vi "Write.vi"(8 "error in":errorcluster, 10 "ConfigData":T1 {"Inactivity Time" format="%#_g Sec"; "Travel Time" format="%#_g Sec"; "Door Close" format="%#_g Sec"; "Door Open" format="%#_g Sec"}, 11 "Config File In":path) -> (0 "error out":errorcluster, 3 "Config File Out":path)   [LabVIEW 2020, in "ConfigurationDatabase.lvlib"]
doc: "Writes and Save configuration data for the simulated configuration database\n[Covers: CD4]"
uses:
  ConfigurationDatabase.lvlib
  Controls/Configuration Data.ctl
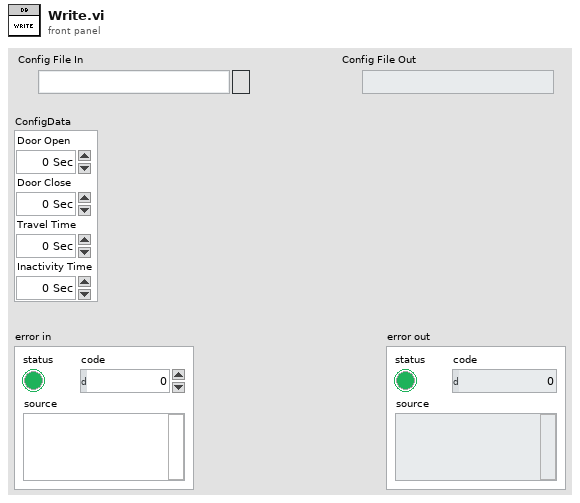
[diagram p1: front panel]
types:
  T1 = typedef "ConfigurationDatabase.lvlib/Configuration Data.ctl" = cluster{"Door Open":dbl, "Door Close":dbl, "Travel Time":dbl, "Inactivity Time":dbl}
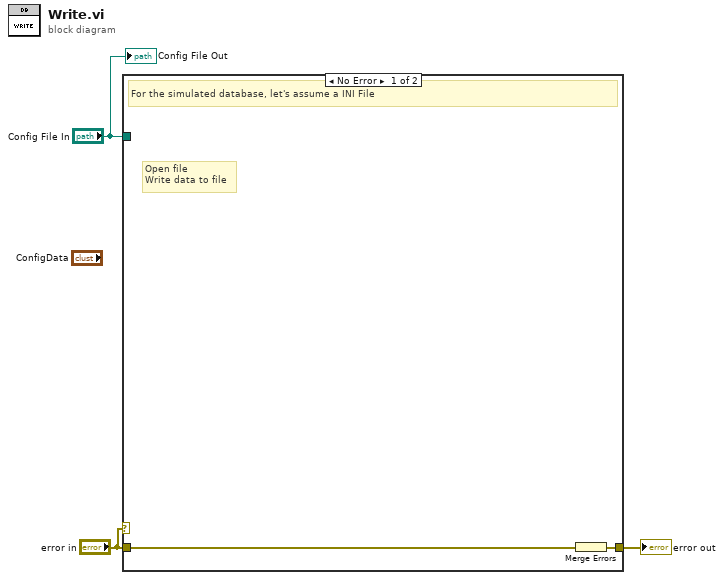
[diagram p0: block diagram]
diagram:
  n1 = case shown="No Error" "error in" {
    tunnel: "error in" -> [w5 w6]
    tunnel: [w4 w6] -> w2
    tunnel: "Config File In" -> [_ _]
    frame No Error {
      # "Open file\nWrite data to file"
      # "For the simulated database, let's assume a INI File"
      n2 = Merge Errors(w5) -> (w4:errorcluster)
    }
    frame Error {
    }
  }
  "error out" <- w2
  "Config File Out" <- "Config File In"
